vi "TCP multi close.vi"(0 "TCP Ports":refnum<k5>[](array[refnum])) -> ()   [LabVIEW 2013]
panel:
  out "Close Errors":errorcluster[](array[cluster])
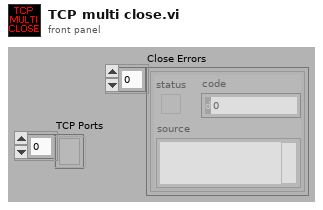
[diagram p1: front panel]
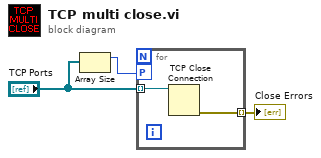
[diagram p0: block diagram]
diagram:
  n1 = Array Size(array="TCP Ports") -> (size(s)=w2:i32)
  n2 = for {
    workers-P: w2 -> [_]
    tunnel: "TCP Ports" -> [w5] mode=indexing
    tunnel: [w4] -> w1 mode=indexing
    n3 = TCP Close Connection(connection ID=w5) -> (error out=w4:errorcluster)  [unwired: 2 in, 1 out]
  }
  "Close Errors" <- w1
